vi "Get Path Loss.vi"(6 "Path Name":string, 8 "error in (no error)":errorcluster, 9 "Frequency (MHz)":u32=600, 10 "Calibration File Name(.ini)":string, 11 "Calibration Root Directory":path) -> (0 "error out":errorcluster, 1 "Not found?":bool, 3 "Path Loss (dB)":dbl)   [LabVIEW 2025]
uses:
  <vilib>/Utility/config.llb/NI_LVConfig.lvlib
  <vilib>/Utility/config.llb/Read Key (String).vi
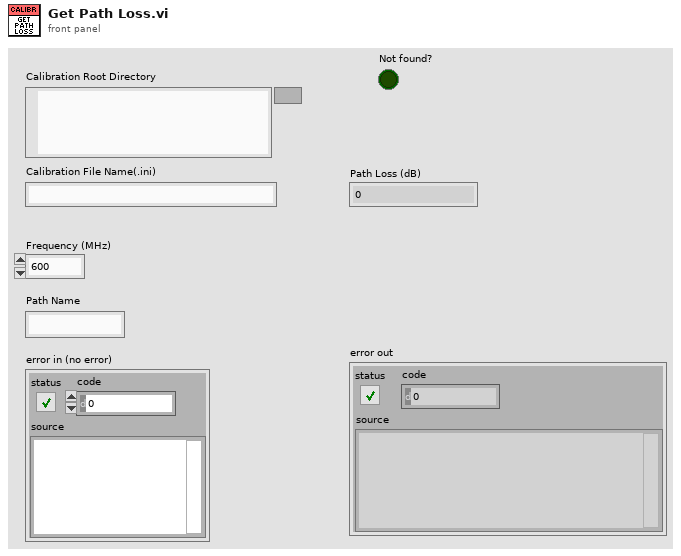
[diagram p1: front panel]
types:
  T1 = typedef "NI_LVConfig.lvlib/Config Data RefNum.ctl" = refnum<k1>
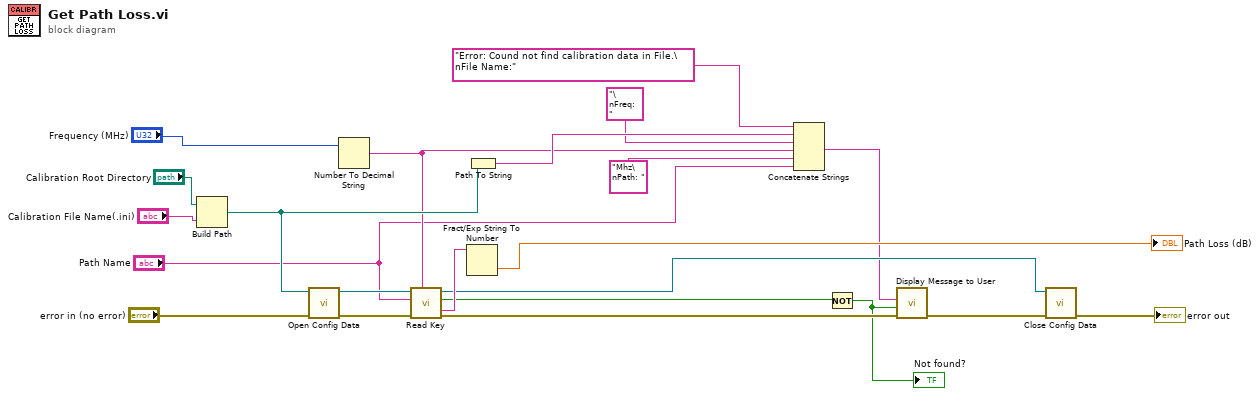
[diagram p0: block diagram]
diagram:
  n1 = Build Path(base path="Calibration Root Directory", name or relative path="Calibration File Name(.ini)") -> (appended path=w8:path)
  n2 = call <vilib>:"Open Config Data.vi"("error in (no error)"="error in (no error)", "configuration file path"=w8) -> ("error out"=w19:errorcluster, "refnum"=w20:T1)  [unwired: 7 in, 1 out]
  n3 = Number To Decimal String(number="Frequency (MHz)") -> (decimal integer string=w4:string)  [unwired: 1 in]
  n4 = call-poly <vilib>:"Read Key.vi"("section"=w4, "error in (no error)"=w19, "key"="Path Name", "refnum"=w20) -> ("error out"=w14:errorcluster, "value"=w18:string, "found?"=w12:bool, "refnum out"=w10:T1)  [unwired: 4 in]
  n5 = Fract/Exp String To Number(string=w18) -> (number=→"Path Loss (dB)":dbl)  [unwired: 3 in, 1 out]
  n6 = Path To String(path=w8) -> (string=w6:string)
  n7 = Concatenate Strings("Error: Cound not find calibration data in File.\nFile Name:", w6, "\nFreq: ", w4, "Mhz\nPath: ", "Path Name") -> (w1:string)
  n8 = Not(x=w12) -> (.not. x?=w11:bool)
  "Not found?" <- w11
  n9 = call "Display Message to User"("error in (no error)"=w14, "Enable"=w11, "Message"=w1) -> ("error out"=w13:errorcluster)  [unwired: 7 in, 1 out]
  n10 = call <vilib>:"Close Config Data.vi"("error in (no error)"=w13, "refnum"=w10) -> ("error out"=→"error out":errorcluster)  [unwired: 8 in, 1 out]
